vi "set IR test parameters.vi"(7 "IR Parameters":T1={"Voltage Level [V]"=500, "Hi Limit [ohm]"=30000000000.0, "Test Time [s] "=8.0, "Dwell Time [s]"=4.4, "Lo Limit [ohm]"=2500000.0, "Ramp Time [s] "=1.1, "Fall Time [s]"=2.2} {"Voltage Level [V]" min=50 max=1000 step=1 format="%.3p"; "Hi Limit [ohm]" min=0.0 max=50000000000000.0 step=100000.0 format="%.1p"; "Test Time [s]" min=0.0 max=999.0 step=0.1 format="%.1p"; "Dwell Time [s]" min=0.0 max=999.0 step=0.1 format="%.1p"; "Lo Limit [ohm]" min=100000.0 max=50000000000000.0 step=100000.0 format="%.1p"; "Ramp Time [s]" min=0.0 max=999.0 step=0.1 format="%.1p"; "Fall Time [s]" min=0.0 max=999.0 step=0.1 format="%.1p"}, 8 "error in (no error)":errorcluster, 10 "Step":T2 min=1 max=99 step=1, 11 "VISA Refnum in":refnum<visa-resource-name>) -> (0 "error out":errorcluster, 3 "VISA Refnum out":refnum<visa-resource-name>)   [LabVIEW 2025]
uses:
  controls/Step--numeric.ctl
  setters & getters/IR parameters--cluster.ctl
  <instrlib>/Chrome 19025/Public/Utility/Type Def/AC-DC-IR modes--ring.ctl
  <instrlib>/Chrome 19025/Public/Utility/Type Def/DC-IR modes--ring.ctl
  <instrlib>/Chrome 19025/Chrome 19025.lvlib
panel:
  # "IR"
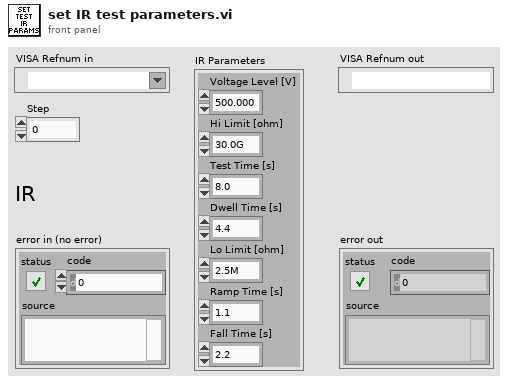
[diagram p1: front panel]
types:
  T1 = typedef "IR parameters--cluster.ctl" = cluster{"Voltage Level [V]":u16, "Hi Limit [ohm]":dbl, "Test Time [s] ":dbl, "Dwell Time [s]":dbl, "Lo Limit [ohm]":dbl, "Ramp Time [s] ":dbl, "Fall Time [s]":dbl}
  T2 = typedef "Step--numeric.ctl" = u8
  T3 = typedef "Chrome 19025.lvlib/DC-IR modes--ring.ctl" = u16
  T4 = typedef "Chrome 19025.lvlib/AC-DC-IR modes--ring.ctl" = u16
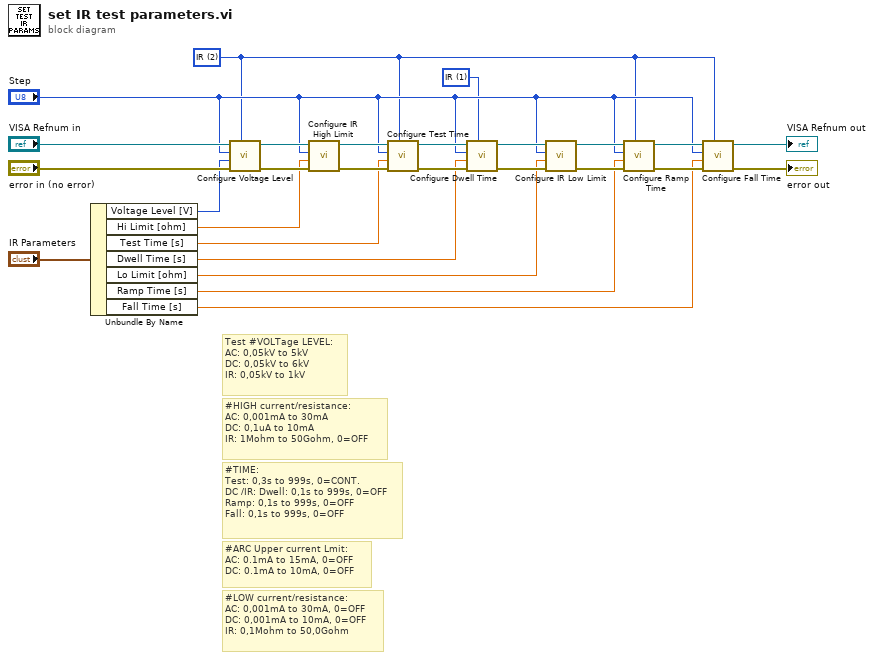
[diagram p0: block diagram]
diagram:
  w10 = T3 1 items=["DC", "IR"] ("Mode")
  w9 = T4 2 items=["AC", "DC", "IR"] ("Mode")
  # "#ARC Upper current Lmit:\nAC: 0.1mA to 15mA, 0=OFF\nDC: 0.1mA to 10mA, 0=OFF"
  # "#TIME: \nTest: 0,3s to 999s, 0=CONT. \nDC /IR: Dwell: 0,1s to 999s, 0=OFF\nRamp: 0,1s to 999s, 0=OFF\nFall: 0,1s to 999s, 0=OFF"
  # "#LOW current/resistance: \nAC: 0,001mA to 30mA, 0=OFF\nDC: 0,001mA to 10mA, 0=OFF\nIR: 0,1Mohm to 50,0Gohm"
  # "#HIGH current/resistance: \nAC: 0,001mA to 30mA\nDC: 0,1uA to 10mA\nIR: 1Mohm to 50Gohm, 0=OFF"
  # "Test #VOLTage LEVEL: \nAC: 0,05kV to 5kV\nDC: 0,05kV to 6kV\nIR: 0,05kV to 1kV"
  n1 = Unbundle By Name("IR Parameters") -> ("Voltage Level [V]"=w7:u16, "Hi Limit [ohm]"=w6:dbl, "Test Time [s]"=w5:dbl, "Dwell Time [s]"=w4:dbl, "Lo Limit [ohm]"=w3:dbl, "Ramp Time [s]"=w2:dbl, "Fall Time [s]"=w1:dbl)
  n2 = call <instrlib>:"Configure Voltage Level.vi"("Mode"=w9, "error in (no error)"="error in (no error)", "Voltage Level [V]"=w7, "Step"="Step", "VISA resource name"="VISA Refnum in") -> ("error out"=w18:errorcluster, "VISA resource name out"=w15:refnum<visa-resource-name>)  [unwired: 5 in]
  n3 = call <instrlib>:"Configure IR High Limit.vi"("error in (no error)"=w18, "Hi Limit [ohm]"=w6, "Step"="Step", "VISA resource name"=w15) -> ("error out"=w21:errorcluster, "VISA resource name out"=w22:refnum<visa-resource-name>)  [unwired: 6 in]
  n4 = call <instrlib>:"Configure Test Time.vi"("Mode"=w9, "error in (no error)"=w21, "Test Time [s]"=w5, "Step"="Step", "VISA resource name"=w22) -> ("error out"=w24:errorcluster, "VISA resource name out"=w12:refnum<visa-resource-name>)  [unwired: 5 in]
  n5 = call <instrlib>:"Configure Dwell Time.vi"("Mode"=w10, "error in (no error)"=w24, "Dwell Time [s]"=w4, "Step"="Step", "VISA resource name"=w12) -> ("error out"=w23:errorcluster, "VISA resource name out"=w25:refnum<visa-resource-name>)  [unwired: 5 in]
  n6 = call <instrlib>:"Configure IR Low Limit.vi"("error in (no error)"=w23, "Low Limit [ohm]"=w3, "Step"="Step", "VISA resource name"=w25) -> ("error out"=w27:errorcluster, "VISA resource name out"=w26:refnum<visa-resource-name>)  [unwired: 6 in]
  n7 = call <instrlib>:"Configure Ramp Time.vi"("Mode"=w9, "error in (no error)"=w27, "Ramp Time [s]"=w2, "Step"="Step", "VISA resource name"=w26) -> ("error out"=w19:errorcluster, "VISA resource name out"=w20:refnum<visa-resource-name>)  [unwired: 5 in]
  n8 = call <instrlib>:"Configure Fall Time.vi"("Mode"=w9, "error in (no error)"=w19, "Fall Time [s]"=w1, "Step"="Step", "VISA resource name"=w20) -> ("error out"=→"error out":errorcluster, "VISA resource name out"=→"VISA Refnum out":refnum<visa-resource-name>)  [unwired: 5 in]
